vi "correlation scan.vi"(1 "Correlations in":cluster{"X":dbl, "Y":dbl}, 5 "Voltages in":cluster{"X":dbl, "Y":dbl}, 6 "Cycle counter":i16, 7 "in put Array":dbl[][](array[numeric]), 8 "T3 positioning \ntest range (V)":T1, 9 "Number of acquisition cycles":i16, 10 "Scanning?":bool) -> (0 "Voltages out":cluster{"X":dbl, "Y":dbl}, 2 "Scanning out":bool, 3 "Output array":dbl[][](array[numeric]), 4 "Cycle counter out":i16)   [LabVIEW 2014]
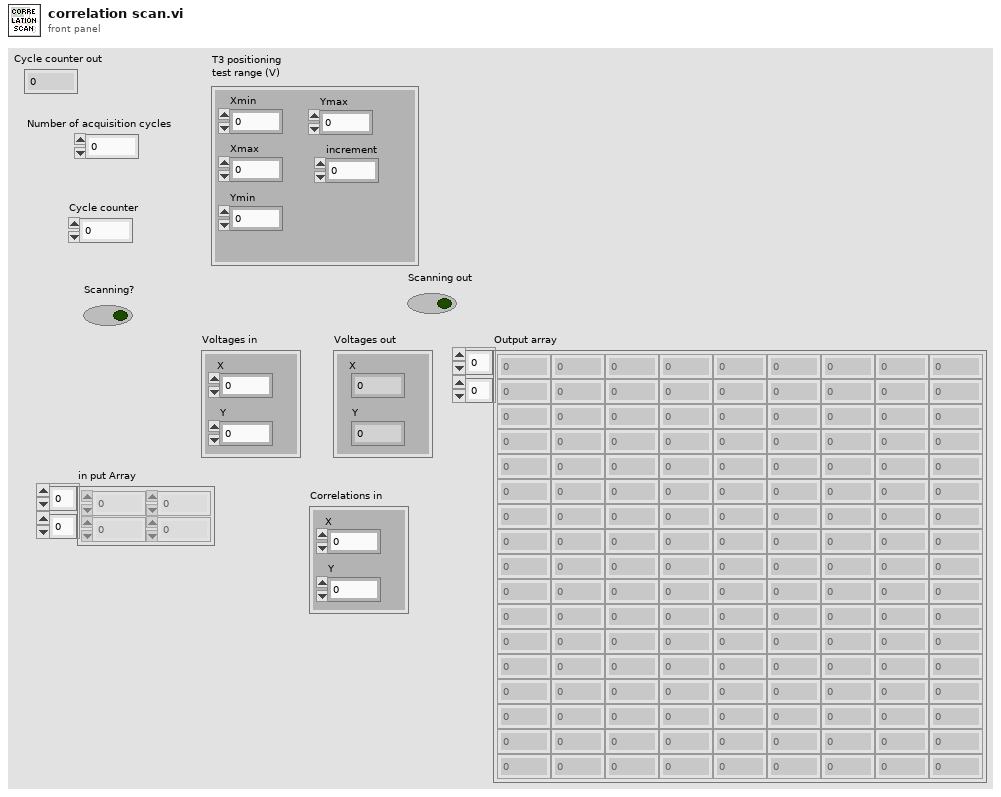
[diagram p1: front panel]
types:
  T1 = cluster{"Xmin":dbl, "Xmax":dbl, "Ymin":dbl, "Ymax":dbl, "increment":dbl}
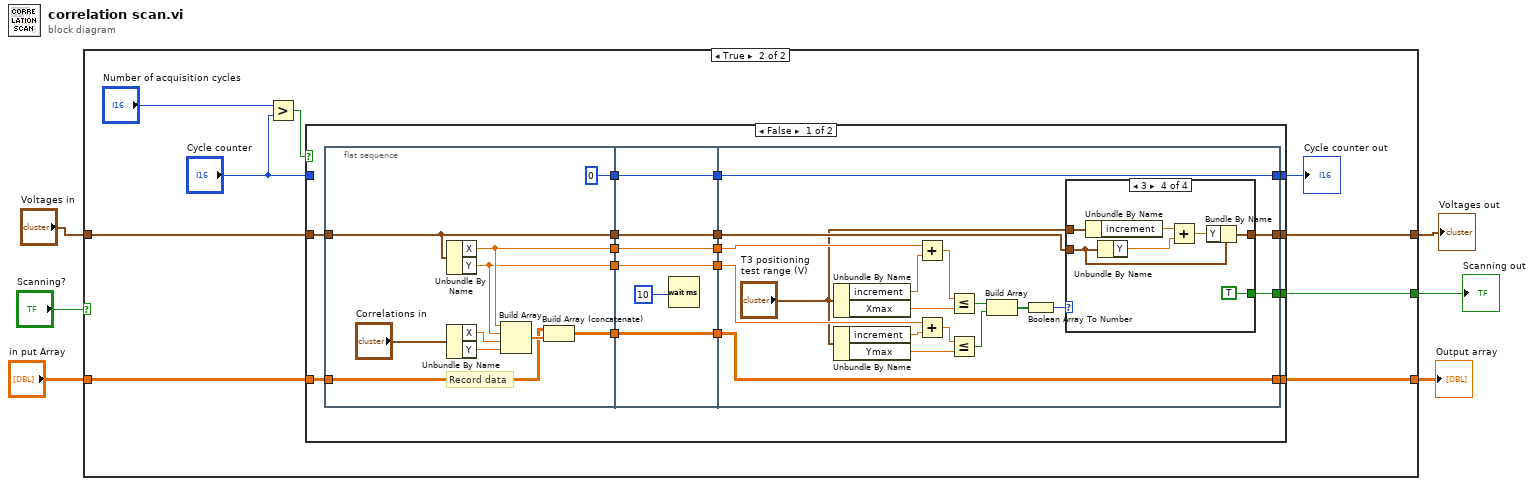
[diagram p0: block diagram]
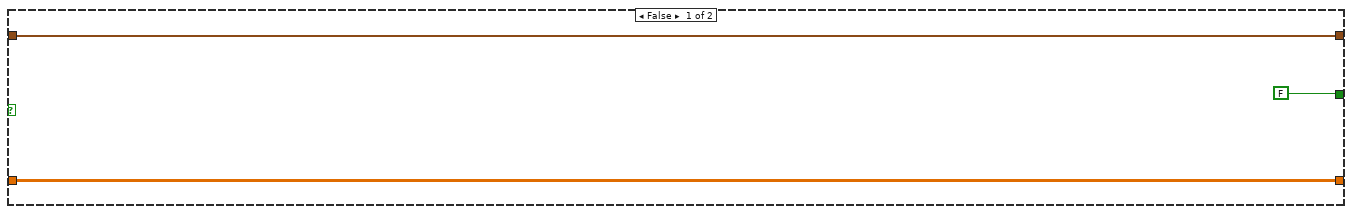
[diagram p2: hidden frame]
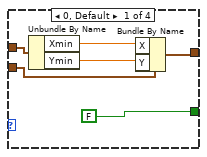
[diagram p3: hidden frame]
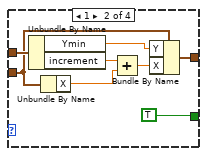
[diagram p4: hidden frame]
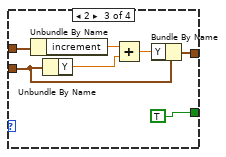
[diagram p5: hidden frame]
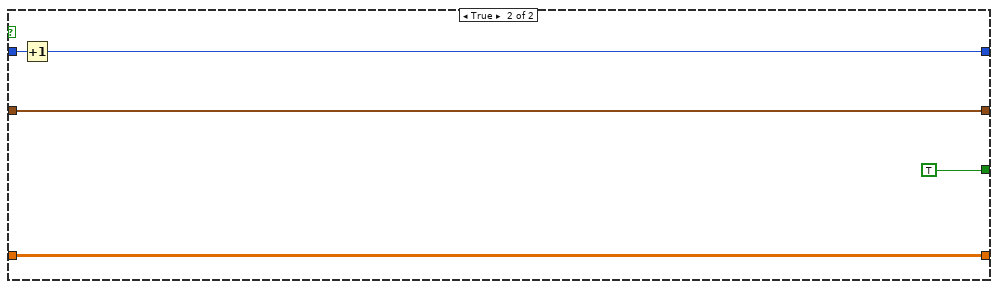
[diagram p6: hidden frame]
diagram:
  n1 = case shown="True" "Scanning?" {
    tunnel: [w9 w14] -> w5
    tunnel: "in put Array" -> [w9 w13]
    tunnel: [FALSE w12] -> w3
    tunnel: [w7 w11] -> w2
    tunnel: "Voltages in" -> [w7 w10]
    frame False {
    }
    frame True {
      n2 = Greater?(x="Number of acquisition cycles", y="Cycle counter") -> (0:w17:bool)
      n3 = case shown="False" w17 {
        tunnel: [w34 w100] -> w16
        tunnel: "Cycle counter" -> [_ w101]
        tunnel: [w33 w99] -> w14
        tunnel: w13 -> [w32 w99]
        tunnel: [w31 TRUE] -> w12
        tunnel: [w30 w97] -> w11
        tunnel: w10 -> [w29 w97]
        frame False {
          n4 = flat-sequence {
            tunnel: w32 -> [w38]
            tunnel: [i16 0] -> w28
            tunnel: [w39] -> w26
            tunnel: [w37] -> w24
            tunnel: [w36] -> w22
            tunnel: [w35] -> w20
            tunnel: w29 -> [w35]
            tunnel: w28 -> [w50]
            tunnel: [w50] -> w27
            tunnel: w26 -> [w49]
            tunnel: [w49] -> w25
            tunnel: w24 -> [w48]
            tunnel: [w48] -> w23
            tunnel: w22 -> [w47]
            tunnel: [w47] -> w21
            tunnel: w20 -> [w46]
            tunnel: [w46] -> w19
            tunnel: [w67] -> w33
            tunnel: [w68] -> w34
            tunnel: w27 -> [w68]
            tunnel: w25 -> [w67]
            tunnel: w23 -> [w66]
            tunnel: w21 -> [w63]
            tunnel: w19 -> [w54]
            tunnel: [w52] -> w30
            tunnel: [w51] -> w31
            frame #0 {
              # "Record data"
              n5 = Unbundle By Name(w35) -> ("X"=w37:dbl, "Y"=w36:dbl)
              n6 = Unbundle By Name("Correlations in") -> ("X"=w42:dbl, "Y"=w41:dbl)
              n7 = Build Array(w37, w36, w42, w41) -> (w40:dbl[])
              n8 = Build Array (concatenate)(w38, w40) -> (w39:dbl[][])
            }
            frame #1 {
              n9 = Wait (ms)(milliseconds to wait=10) -> ()  [unwired: 1 out]
            }
            frame #2 {
              n10 = Unbundle By Name("T3 positioning \ntest range (V)") -> ("increment"=w65:dbl, "Xmax"=w59:dbl)
              n11 = Unbundle By Name("T3 positioning \ntest range (V)") -> ("increment"=w64:dbl, "Ymax"=w61:dbl)
              n12 = Add(x=w66, y=w65) -> (x+y=w60:dbl)
              n13 = Add(x=w63, y=w64) -> (x+y=w62:dbl)
              n14 = Less Or Equal?(x=w60, y=w59) -> (x <= y?=w58:bool)
              n15 = Less Or Equal?(x=w62, y=w61) -> (x <= y?=w57:bool)
              n16 = Build Array(w58, w57) -> (w56:bool[])
              n17 = Boolean Array To Number(Boolean array=w56) -> (number=w55:u32)
              n18 = case shown="3" w55 {
                tunnel: w54 -> [w73 w79 w86 w96]
                tunnel: "T3 positioning \ntest range (V)" -> [w74 w82 w85 w94]
                tunnel: [w70 w76 w84 w91] -> w52
                tunnel: [FALSE TRUE TRUE TRUE] -> w51
                frame 0, Default {
                  n19 = Unbundle By Name(w74) -> ("Xmin"=w72:dbl, "Ymin"=w71:dbl)
                  n20 = Bundle By Name(cluster=w73, "X"=w72, "Y"=w71) -> (w70:cluster{"X":dbl, "Y":dbl})
                }
                frame 1 {
                  n21 = Unbundle By Name(w82) -> ("Ymin"=w78:dbl, "increment"=w81:dbl)
                  n22 = Unbundle By Name(w79) -> ("X"=w80:dbl)
                  n23 = Add(x=w81, y=w80) -> (x+y=w77:dbl)
                  n24 = Bundle By Name(cluster=w79, "Y"=w78, "X"=w77) -> (w76:cluster{"X":dbl, "Y":dbl})
                }
                frame 2 {
                  n25 = Unbundle By Name(w85) -> ("increment"=w88:dbl)
                  n26 = Unbundle By Name(w86) -> ("Y"=w89:dbl)
                  n27 = Add(x=w88, y=w89) -> (x+y=w87:dbl)
                  n28 = Bundle By Name(cluster=w86, "Y"=w87) -> (w84:cluster{"X":dbl, "Y":dbl})
                }
                frame 3 {
                  n29 = Unbundle By Name(w94) -> ("increment"=w93:dbl)
                  n30 = Unbundle By Name(w96) -> ("Y"=w95:dbl)
                  n31 = Add(x=w93, y=w95) -> (x+y=w92:dbl)
                  n32 = Bundle By Name(cluster=w96, "Y"=w92) -> (w91:cluster{"X":dbl, "Y":dbl})
                }
              }
            }
          }
        }
        frame True {
          n33 = Increment(x=w101) -> (x+1=w100:i16)
        }
      }
      "Cycle counter out" <- w16
    }
  }
  "Output array" <- w5
  "Scanning out" <- w3
  "Voltages out" <- w2
